vi "TRIG_CHAN_AUX_POS.vi"(0 "VISA IN":refnum<visa-resource-name>, 1 "Aux":i32, 2 "Position":string(combo)="BEF", 5 "error in":errorcluster, 7 "Channel":i32) -> (14 "VISA Out":refnum<visa-resource-name>, 19 "error out":errorcluster)   [LabVIEW 2018, in "PNA-X.lvlib"]
doc: "TRIGger:CHANnel<ch>:AUX<n>:POSition <char> \n1891\n\n(Read-Write) Specifies whether the aux trigger out signal is sent BEFore or AFTer the acquisition. \nParameters \n<ch> Any existing channel number. If unspecified, value is set to 1. \n<n> Rear panel connector used to send or receive signals. \nPNA-X - choose from 1 (AUX TRIG 1) or 2 (AUX TRIG 2) \nAll other models: choose 1. (BNC Trig I/O \nIf unspecified, value is set to 1. \n<char> Choose from: \nBEFore Use if the external device needs to be triggered before the data is \nacquired, such as a power meter. \nAFTer Use if the external device needs to be triggered just after data has been \nacquired, such as an external source. This could be more efficient since it allows \nthe external device to get ready for the next acquisition at the same time as the \nPNA. \nExamples TRIG:CHAN:AUX:POS BEF \ntrigger:channel2:aux2:position after \nQuery Syntax TRIGger:CHANnel<ch>:AUX<n>:POSition? \nReturn Type Character \nDefault AFTer"
uses:
  PNA-X.lvlib
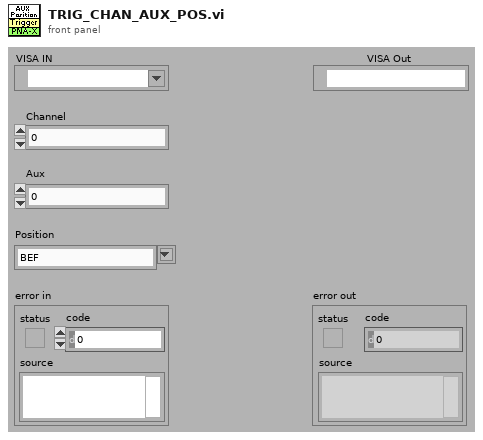
[diagram p1: front panel]
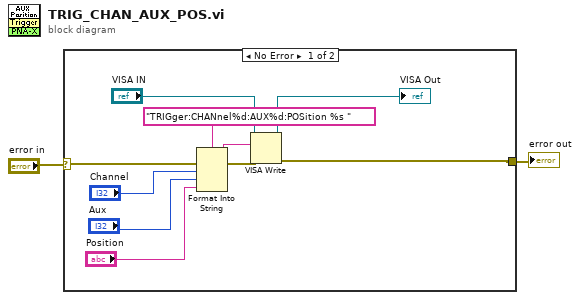
[diagram p0: block diagram]
diagram:
  n1 = case shown="No Error" "error in" {
    selector: "error in" -> [w12 w13]
    tunnel: [w7 w13] -> w1
    frame No Error {
      n2 = Format Into String(format string="TRIGger:CHANnel%d:AUX%d:POSition %s " ("Cmdline"), error in=w12, "Channel", "Aux", "Position") -> (resulting string=w10:string, error out=w11:errorcluster)  [unwired: 1 in]
      n3 = VISA Write(VISA resource name="VISA IN", write buffer=w10, error in (no error)=w11) -> (VISA resource name out=→"VISA Out":refnum<visa-resource-name>, error out=w7:errorcluster)  [unwired: 1 out]
    }
    frame Error {
    }
  }
  "error out" <- w1
